vi "Day of the Week Predictor.vi"(6 "EXIT":bool, 7 "Guess the Day":bool, 8 "error in":errorcluster, 9 "YEAR\n(0-2399)A.D":i32, 10 "DATE":u16(ring) items=["1", "2", "3", "4", "5", "6", "7", "8", "9", "10", "11", "12", "13", "14", "15", "16", "17", "18", "19", "20", "21", "22", "23", "24", "25", "26", "27", "28", "29", "30", "31"], 11 "MONTH":T1(ring)) -> (0 "error out":errorcluster)   [LabVIEW 2020]
doc: "This VI will predict the Day of the Week from a given set of years (0-2399) A.D.\nUser can set the Month,Date,Year and then Click the \"GUESS THE DAY\" button to get the Day from given details."
uses:
  <vilib>/regexp/Match Regular Expression.xnode
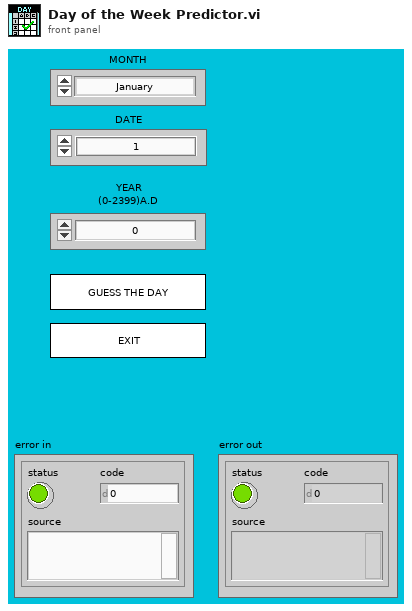
[diagram p1: front panel]
types:
  T1 = enum16{"January", "February", "March", "April", "May", "June", "July", "August", "September", "October", "November", "December"}
  T2 = enum32{"Invalid", "Standard", "Closed", "Hidden", "Minimized", "Maximized"}
  T3 = enum32{"invalid app kind", "Development System", "Run Time System", "Student Edition", "Embedded LabVIEW", "Evaluation", "Custom"}
  T4 = cluster{"Core":cluster{"Current VI Reference":refnum<vi>, "Close Panel on Exit?":bool}, "Your Boolean data":bool, "Your string data":string, "Year":i32, "Month":enum16{"January", "February", "March", "April", "May", "June", "July", "August", "September", "October", "November", "December"}, "Date":enum16{"1", "2", "3", "4", "5", "6", "7", "8", "9", "10", "11", "12", "13", "14", "15", "16", "17", "18", "19", "20", "21", "22", "23", "24", "25", "26", "27", "28", "29", "30", "31"}, "Last two Digits(Year)":i32, "Quotient(/4)":i32, "Month Code":i32, "Year Code":i32}
  T5 = enum16{"1", "2", "3", "4", "5", "6", "7", "8", "9", "10", "11", "12", "13", "14", "15", "16", "17", "18", "19", "20", "21", "22", "23", "24", "25", "26", "27", "28", "29", "30", "31"}
  T6 = cluster{"Current VI Reference":refnum<vi>, "Close Panel on Exit?":bool}
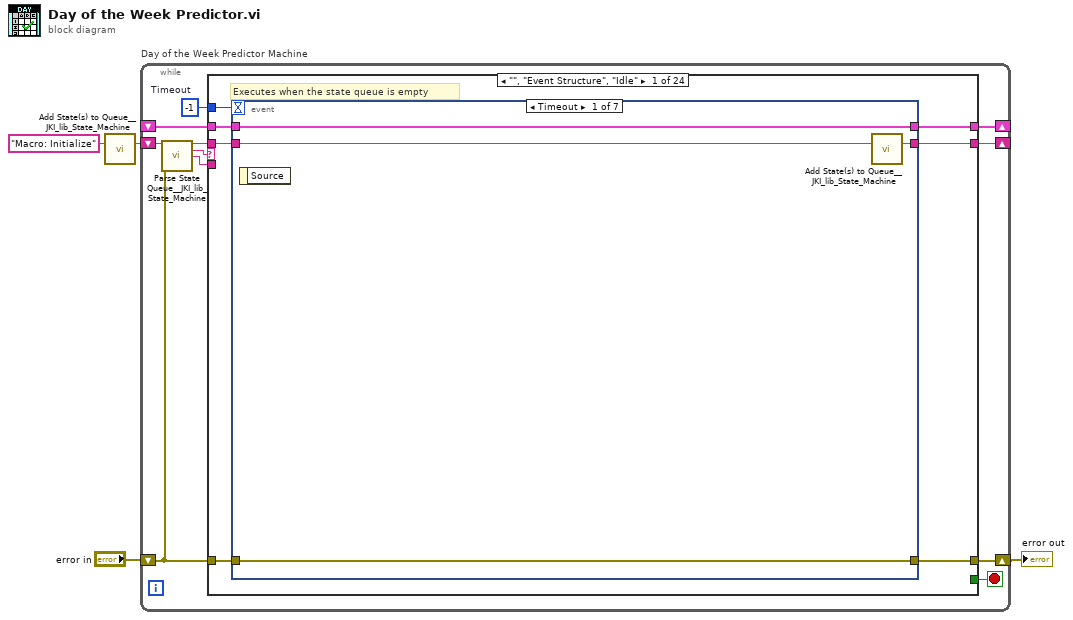
[diagram p0: block diagram]
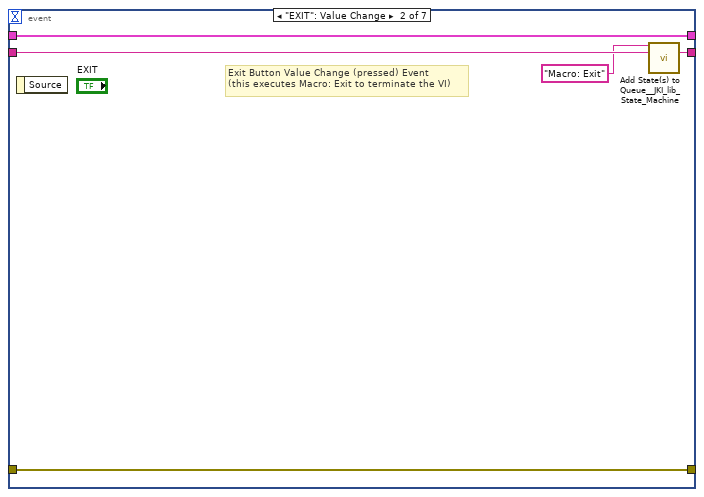
[diagram p2: hidden frame]
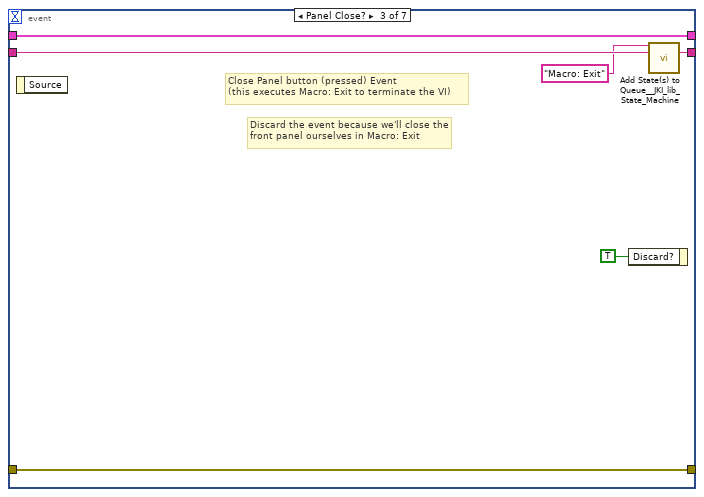
[diagram p3: hidden frame]
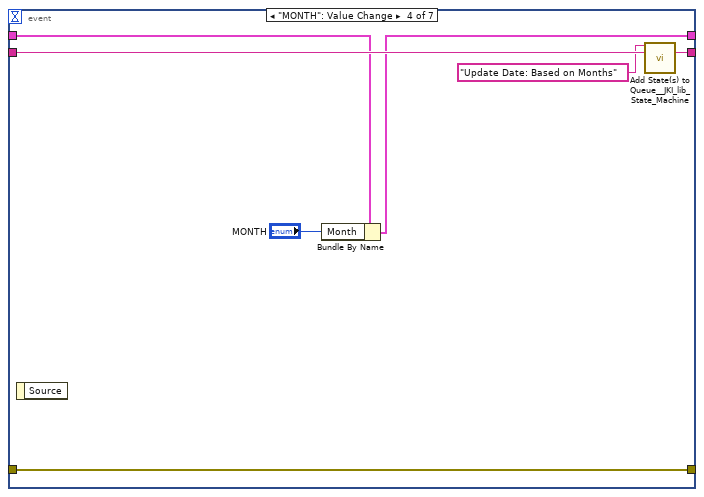
[diagram p4: hidden frame]
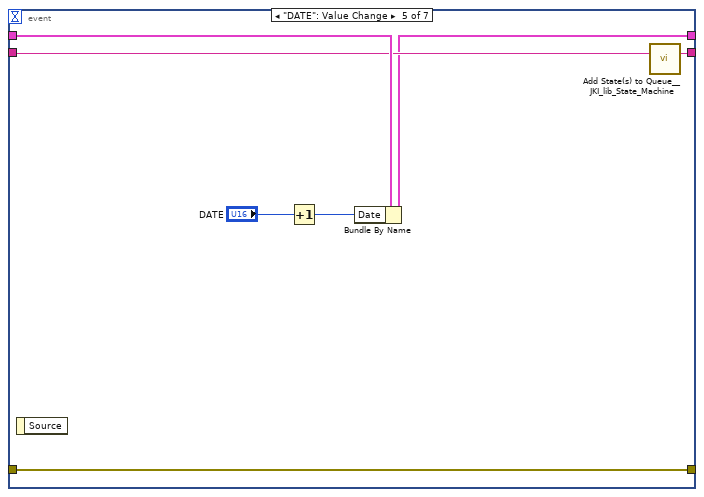
[diagram p5: hidden frame]
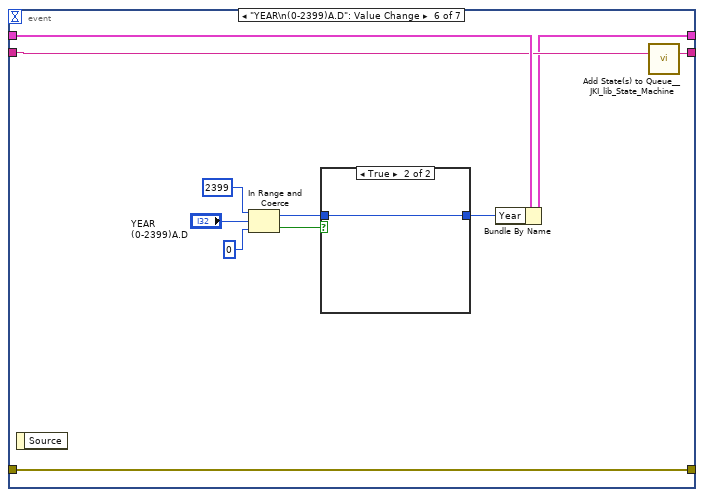
[diagram p6: hidden frame]
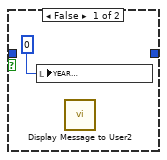
[diagram p7: hidden frame]
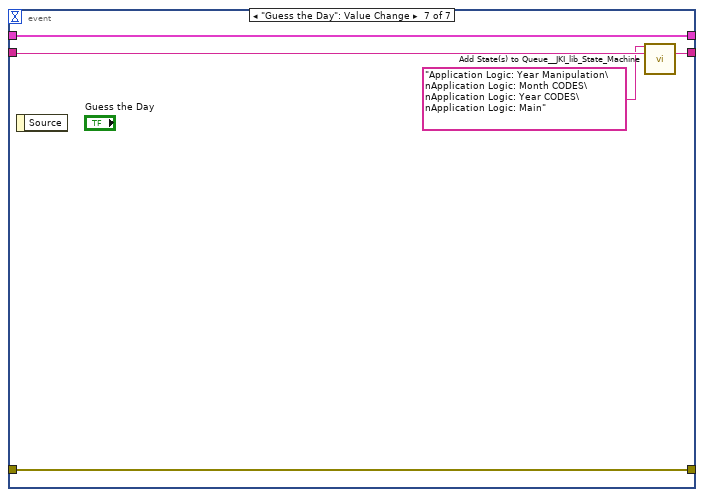
[diagram p8: hidden frame]
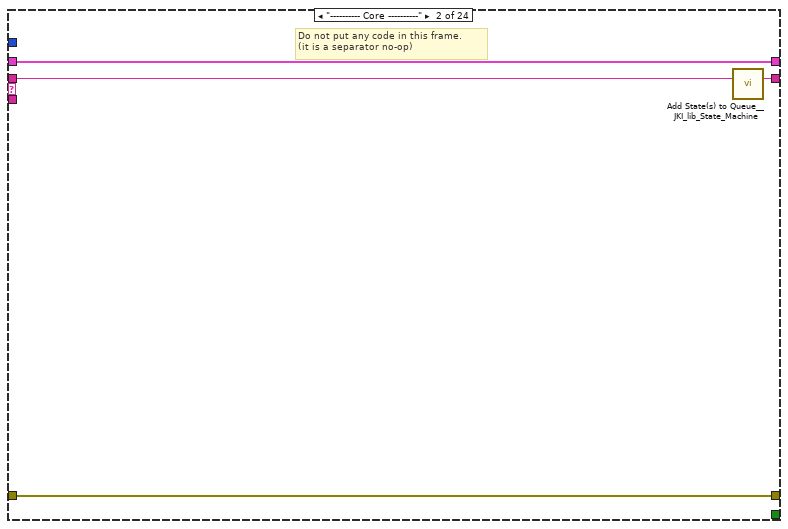
[diagram p9: hidden frame]
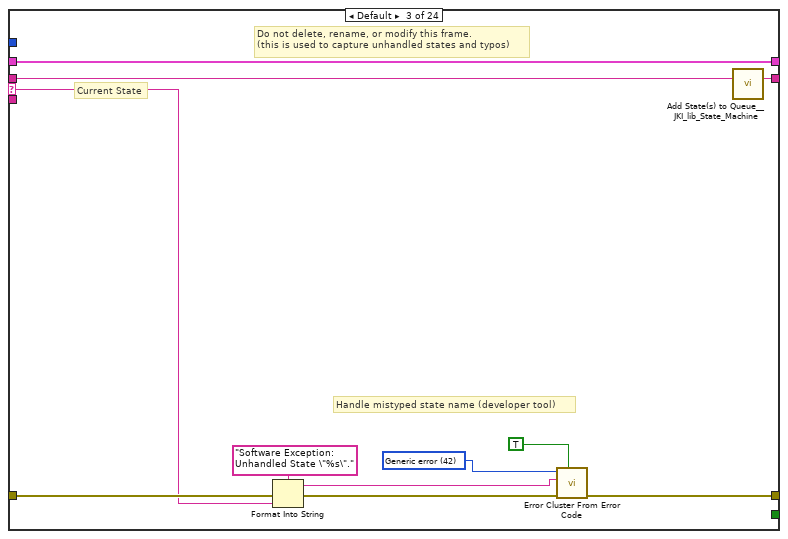
[diagram p10: hidden frame]
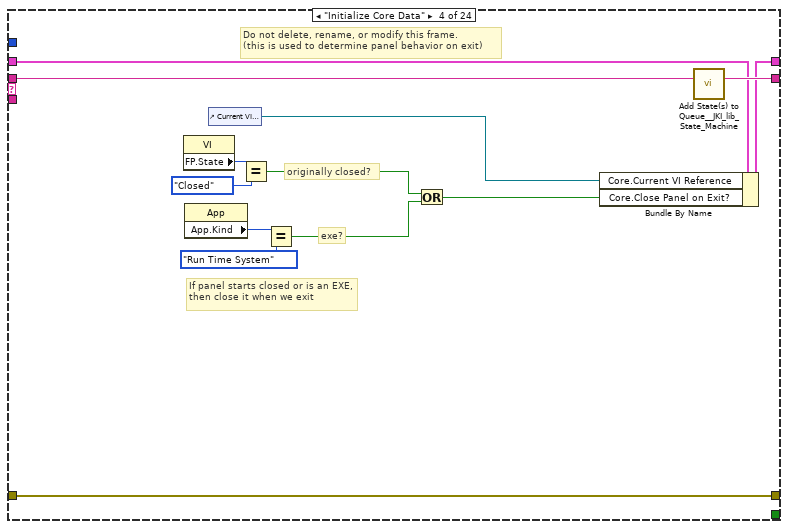
[diagram p11: hidden frame]
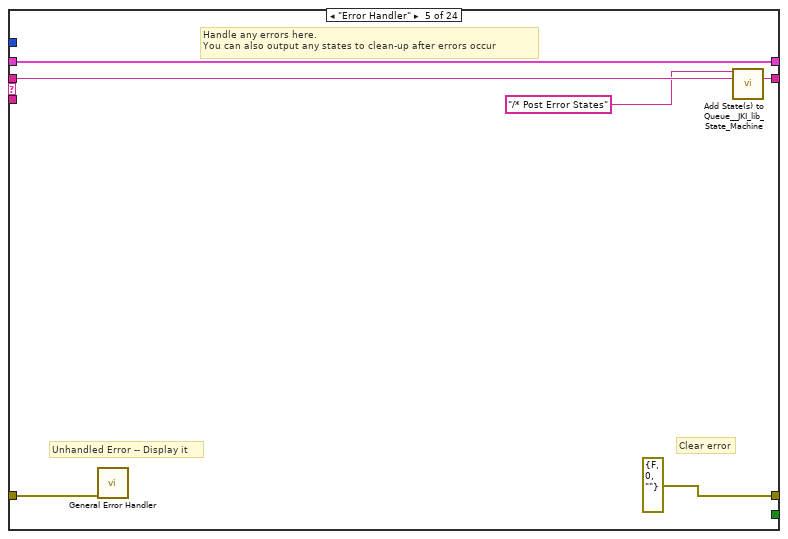
[diagram p12: hidden frame]
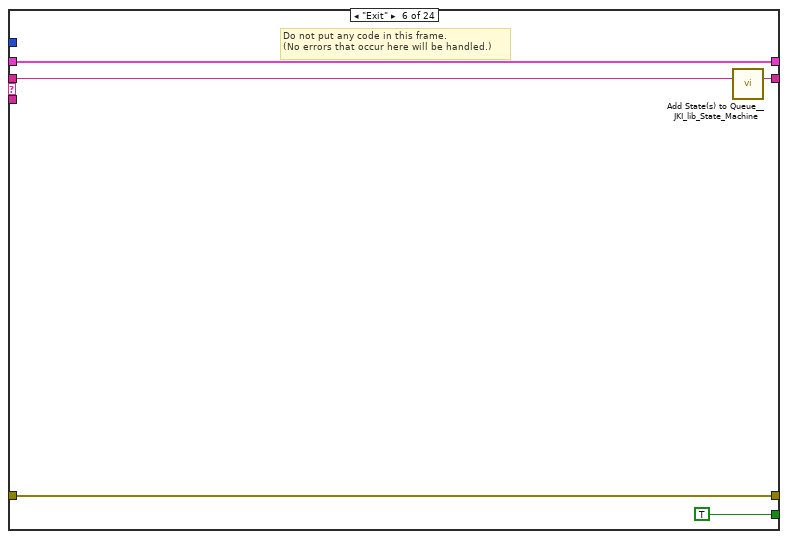
[diagram p13: hidden frame]
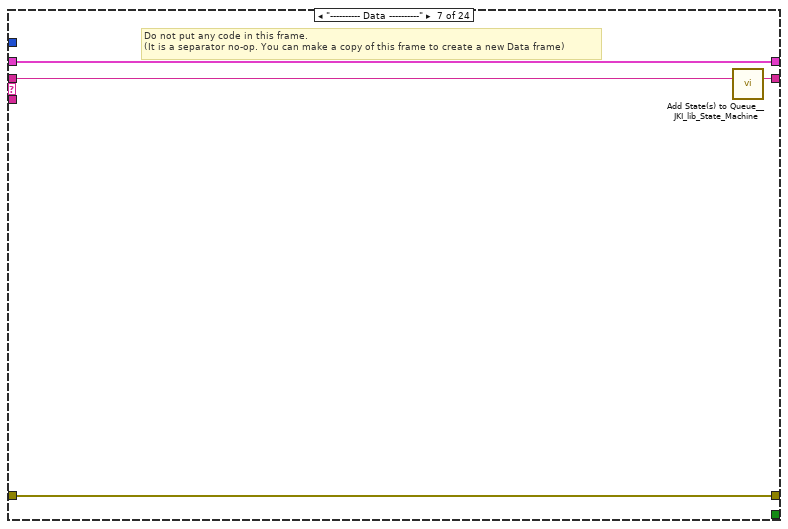
[diagram p14: hidden frame]
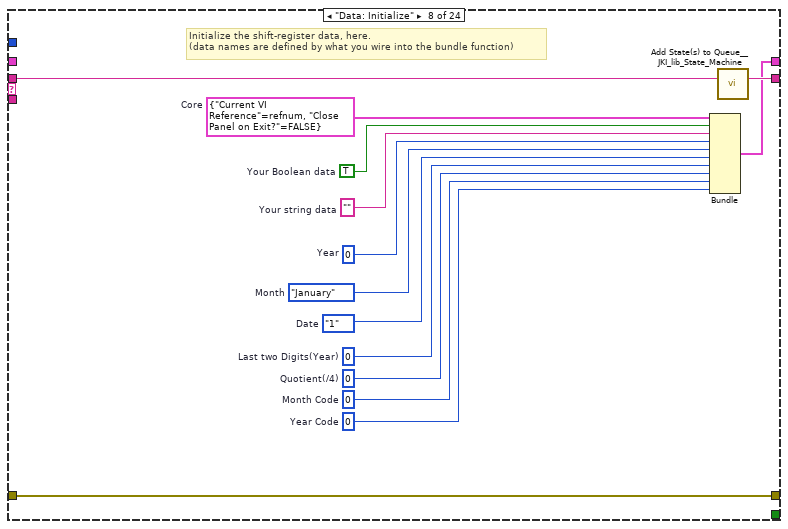
[diagram p15: hidden frame]
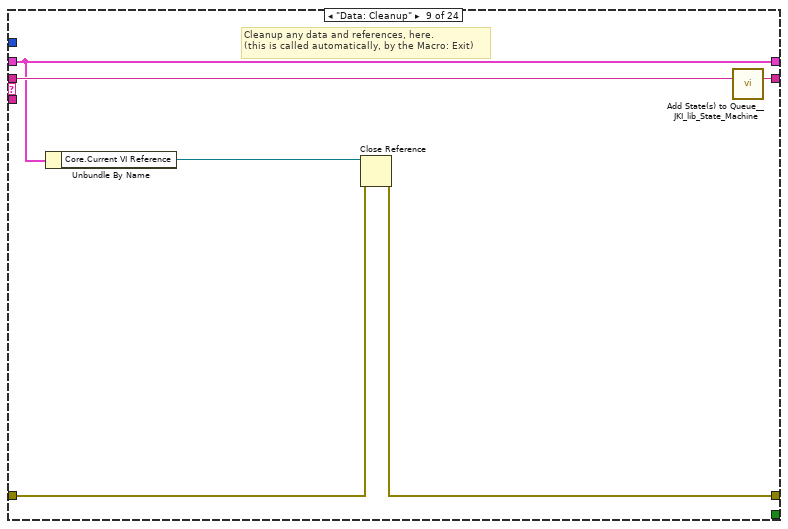
[diagram p16: hidden frame]
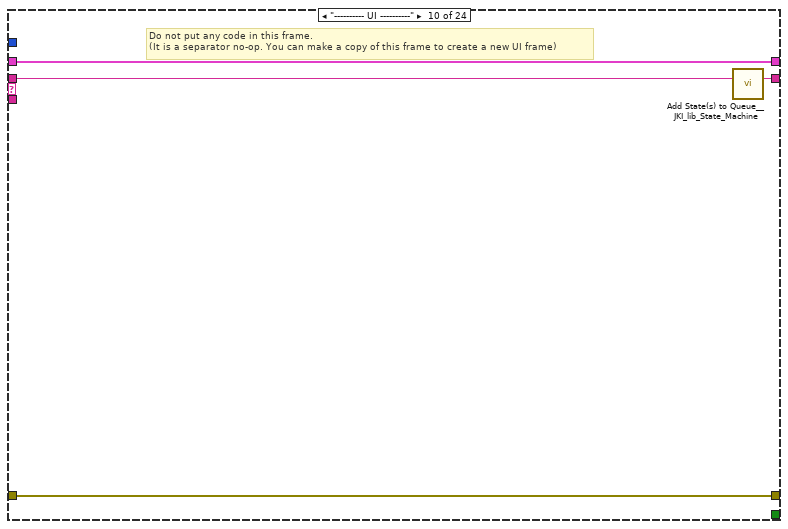
[diagram p17: hidden frame]
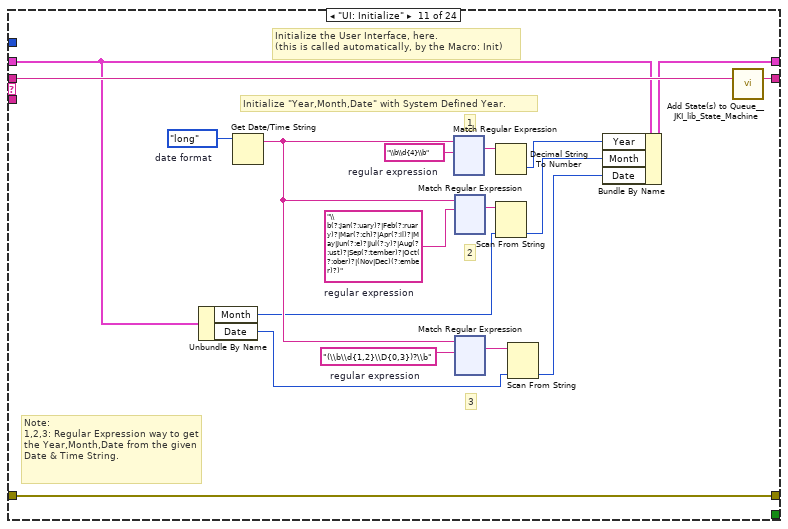
[diagram p18: hidden frame]
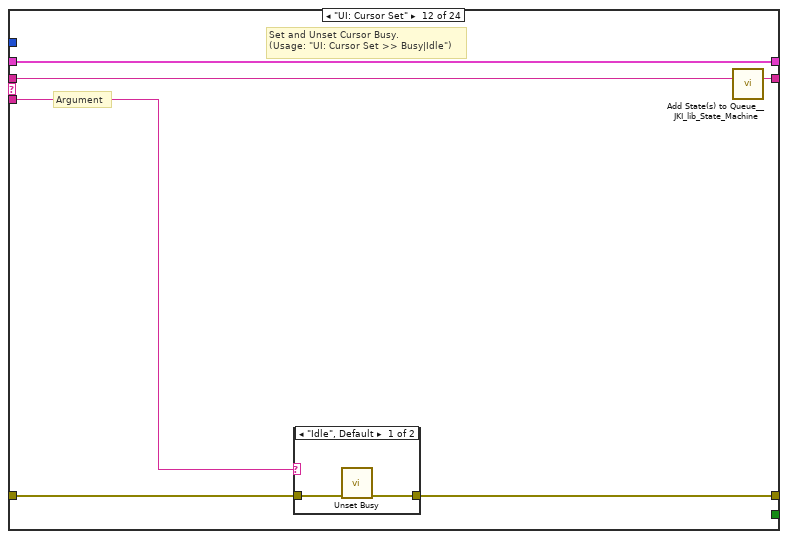
[diagram p19: hidden frame]
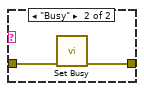
[diagram p20: hidden frame]
diagram:
  n1 = call <vilib>:"Add State(s) to Queue__JKI_lib_State_Machine.vi"("State(s) in (\"\")"="Macro: Initialize") -> ("States Out"=w4:string)  [unwired: 14 in]
  n2 = while "Day of the Week Predictor Machine" {
    shift-right: [w8] -> _
    shift-left: _ -> [w7]
    shift-right: [w11] -> w1
    shift-left: "error in" -> [w5]
    shift-right: [w10] -> _
    shift-left: w4 -> [w12]
    stop <- w9 stop-if-true
    w6 = -1  # Timeout
    n3 = call <vilib>:"Parse State Queue__JKI_lib_State_Machine.vi"("State Queue"=w12, "Error In (no error)"=w5) -> ("Remaining States"=w14:string, "Current State"=w15:string, "Arguments"=w13:string)  [unwired: 11 in]
    n4 = case shown="\"\", \"Event Structure\", \"Idle\"" w15 {
      selector: w15 -> [_ _ w74 _ _ _ _ _ _ _ _ _ _ _ _ _ _ _ _ _ _ _ _ _]
      tunnel: w14 -> [w22 w73 w78 w97 w103 w108 w112 w126 w132 w136 w154 w502 w513 w585 w589 w594 w604 w608 w616 w632 w645 w663 w670 w690]
      tunnel: w13 -> [_ _ _ _ _ _ _ _ _ _ _ w497 w507 _ _ _ _ _ _ _ _ _ _ _]
      tunnel: w7 -> [w20 w70 w76 w90 w100 w106 w109 _ w127 w133 w140 w500 w509 w582 w586 w591 w601 w605 w613 w629 w642 w660 w667 w687]
      tunnel: [w19 w71 w80 w94 errorcluster {"status"=FALSE, "code"=0, "source"=""} ("error out") w105 w110 w123 w128 w134 w152 w498 w510 w583 w587 w592 w602 w606 w614 w630 w643 w661 w668 w688] -> w11
      tunnel: w5 -> [w18 w71 w79 w94 w99 w105 w110 w123 w129 w134 w152 w499 w511 w583 w587 w592 w602 w606 w614 w630 w643 w661 w668 w688]
      tunnel: [w21 w72 w77 w96 w102 w107 w111 w125 w131 w135 w153 w501 w512 w584 w588 w593 w603 w607 w615 w631 w644 w662 w669 w689] -> w10
      tunnel: [_ _ _ _ _ TRUE _ _ _ _ _ _ _ _ _ _ _ _ _ _ _ _ _ _] -> w9
      tunnel: [w17 w70 w76 w95 w100 w106 w109 w124 w127 w133 w148 w500 w509 w582 w586 w591 w601 w605 w613 w629 w642 w656 w665 w685] -> w8
      tunnel: w6 -> [w16 _ _ _ _ _ _ _ _ _ _ _ _ _ _ _ _ _ _ _ _ _ _ _]
      frame "", "Event Structure", "Idle" {
        # "Executes when the state queue is empty"
        n5 = event shown="[0] Timeout" {
          selector: _ -> [_ _ _ _ _ _ _]
          dyn-events: _ -> [_ _ _ _ _ _ _]
          timeout: w16 -> [_ _ _ _ _ _ _]
          tunnel: w22 -> [w26 w31 w37 w43 w49 w59 w66]
          tunnel: [w25 w30 w36 w44 w50 w60 w67] -> w21
          tunnel: w20 -> [w23 w28 w34 w41 w51 w62 w68]
          tunnel: [w24 w29 w35 w38 w47 w61 w69] -> w19
          tunnel: w18 -> [w24 w29 w35 w38 w47 w61 w69]
          tunnel: [w23 w28 w34 w40 w48 w58 w68] -> w17
          event Timeout {
            n6 = event-data() -> ()  [unwired: 1 in, 1 out]
            n7 = call <vilib>:"Add State(s) to Queue__JKI_lib_State_Machine.vi"("State(s) in (\"\")"=w26) -> ("States Out"=w25:string)  [unwired: 14 in]
          }
          event "EXIT": Value Change {
            # "Exit Button Value Change (pressed) Event\n(this executes Macro: Exit to terminate the VI)"
            n8 = event-data() -> ()  [unwired: 1 in, 1 out]
            n9 = call <vilib>:"Add State(s) to Queue__JKI_lib_State_Machine.vi"("State(s) in Front (\"\")"="Macro: Exit", "State(s) in (\"\")"=w31) -> ("States Out"=w30:string)  [unwired: 13 in]
          }
          event Panel Close? {
            # "Discard the event because we'll close the front panel ourselves in Macro: Exit"
            # "Close Panel button (pressed) Event\n(this executes Macro: Exit to terminate the VI)"
            n10 = event-data() -> ()  [unwired: 1 in, 1 out]
            n11 = event-data("Discard?"=TRUE) -> ()  [unwired: 1 in, 1 out]
            n12 = call <vilib>:"Add State(s) to Queue__JKI_lib_State_Machine.vi"("State(s) in Front (\"\")"="Macro: Exit", "State(s) in (\"\")"=w37) -> ("States Out"=w36:string)  [unwired: 13 in]
          }
          event "MONTH": Value Change {
            n13 = event-data() -> ()  [unwired: 1 in, 1 out]
            n14 = Bundle By Name(cluster=w41, "Month"="MONTH") -> (w40:T4)
            n15 = call <vilib>:"Add State(s) to Queue__JKI_lib_State_Machine.vi"("State(s) in Front (\"\")"="Update Date: Based on Months", "State(s) in (\"\")"=w43) -> ("States Out"=w44:string)  [unwired: 13 in]
          }
          event "DATE": Value Change {
            n16 = event-data() -> ()  [unwired: 1 in, 1 out]
            n17 = Increment(x="DATE") -> (x+1=w45:u16)
            n18 = Bundle By Name(cluster=w51, "Date"=w45) -> (w48:T4)
            n19 = call <vilib>:"Add State(s) to Queue__JKI_lib_State_Machine.vi"("State(s) in (\"\")"=w49) -> ("States Out"=w50:string)  [unwired: 14 in]
          }
          event "YEAR\n(0-2399)A.D": Value Change {
            n20 = event-data() -> ()  [unwired: 1 in, 1 out]
            n21 = In Range and Coerce(upper limit=2399, x="YEAR\n(0-2399)A.D", lower limit=0) -> (coerced(x)=w53:i32, In Range?=w54:bool)
            n22 = case shown="True" w54 {
              tunnel: [_ w64] -> w52
              tunnel: w53 -> [_ w64]
              frame False {
                n23 = local write "YEAR\n(0-2399)A.D"(0 ("YEAR\n(0-2399)A.D")) -> ()
                n24 = call "Display Message to User2"() -> ()  [unwired: 10 in, 2 out]
              }
              frame True {
              }
            }
            n25 = Bundle By Name(cluster=w62, "Year"=w52) -> (w58:T4)
            n26 = call <vilib>:"Add State(s) to Queue__JKI_lib_State_Machine.vi"("State(s) in (\"\")"=w59) -> ("States Out"=w60:string)  [unwired: 14 in]
          }
          event "Guess the Day": Value Change {
            n27 = event-data() -> ()  [unwired: 1 in, 1 out]
            n28 = call <vilib>:"Add State(s) to Queue__JKI_lib_State_Machine.vi"("State(s) in Front (\"\")"="Application Logic: Year Manipulation\nApplication Logic: Month CODES\nApplication Logic: Year CODES\nApplication Logic: Main" ("State(s) in (\"\")"), "State(s) in (\"\")"=w66) -> ("States Out"=w67:string)  [unwired: 13 in]
          }
        }
      }
      frame "---------- Core ----------" {
        # "Do not put any code in this frame.\n(it is a separator no-op)"
        n29 = call <vilib>:"Add State(s) to Queue__JKI_lib_State_Machine.vi"("State(s) in (\"\")"=w73) -> ("States Out"=w72:string)  [unwired: 14 in]
      }
      frame Default {
        w83 = 42 items=["No error", "Argument error", "Memory is full", "Out of zone", "End of file", "File already open", "Generic file I/O error", "File not found", "File permission error", "Disk is full", "Duplicate path", "Too many files open", "System feature not enabled", "Resource file not found", "Cannot add resource", "Resource not found", "Image not found", "Image memory error", "Pen does not exist", "Config type invalid", "Config token not found", "Config parse error", "Config memory error", "Bad external code format", "Bad external code offset", "External code not present", "Null window", "Destroy window error", "Null menu", "Print aborted", "Bad print record", "Print driver error", "Windows error during printing", "Memory error during printing", "Print dialog error", "Generic print error", "Invalid device refnum", "Device not found", "Device parameter error", "Device unit error", "Cannot open device", "Device call aborted", "Generic error", "Cancelled by user", "Object ID too low", "Object ID too high", "Object not in heap", "Unknown heap", "Unknown object (invalid DefProc)", "Unknown object (DefProc not in table)", "Message out of range", "Invalid (null) method", "Unknown message", "Manager call not supported", "Bad address", "Network operation in progress", "Network operation timed out", "Connection is busy", "Network attribute not supported", "Network error", "Address in use", "System out of memory", "Connection aborted", "Connection refused", "Not connected", "Already connected", "Connection closed", "Initialization error (interapplication manager)", "Bad occurrence", "Wait on unbound occurrence handler", "Occurrence queue overflow", "Datalog type conflict", "Unused", "Unrecognized type (interapplication manager)", "Memory corrupt", "Failed to make temporary DLL", "Old CIN version", "Drag socket not found", "Failed to load drop-object", "Failed to register OLE object", "Failed to release OLE object", "Format specifier type mismatch", "Unknown format specifier", "Too few format specifiers", "Too many format specifiers", "Scan failed", "Newer CIN version", "Error converting to variant", "Runtime menu error", "Password tampered", "Variant attribute not found", "Incompatible variant data type", "Event data is not available", "Event Store is not present", "Occurrence is not found", "Event Queue is not created", "Event info is not available", "Refnum passed is NULL", "Error retrieving Class GUID", "Error retrieving CoClass GUID", "Error retrieving TypeLib GUID.", "Bad built application magic bytes.", "Specific driver is different from the specific driver associated with the Logical Name.", "There is no session opened to the class driver.", "Max Error", "MAX - Error with config objects", "MAX - Error loading configuration", "MAX - Group not supported"]
        # "Current State"
        # "Do not delete, rename, or modify this frame.\n(this is used to capture unhandled states and typos)"
        # "Handle mistyped state name (developer tool)"
        n30 = Format Into String(format string="Software Exception: Unhandled State \"%s\"." ("message"), error in=w79, w74) -> (resulting string=w82:string, error out=w81:errorcluster)  [unwired: 1 in]
        n31 = call <vilib>:"Error Cluster From Error Code.vi"("show call chain? (False)"=TRUE, "error in (no error)"=w81, "error message (\"\")"=w82, "error code (0)"=w83) -> ("error out"=w80:errorcluster)  [unwired: 5 in]
        n32 = call <vilib>:"Add State(s) to Queue__JKI_lib_State_Machine.vi"("State(s) in (\"\")"=w78) -> ("States Out"=w77:string)  [unwired: 14 in]
      }
      frame "Initialize Core Data" {
        # "Do not delete, rename, or modify this frame.\n(this is used to determine panel behavior on exit)"
        # "originally closed?"
        # "exe?"
        # "If panel starts closed or is an EXE, then close it when we exit"
        n33 = property class="VI"() -> ("FP.State"=w87:T2)  [unwired: 2 in, 2 out]
        n34 = property class="App"() -> ("App.Kind"=w93:T3)  [unwired: 2 in, 2 out]
        n35 = control-ref of="Current VI Reference"() -> (w88:refnum<vi>)
        n36 = Equal?(x=w87, y=T2."Closed" ("Front Panel Window:State")) -> (x = y?=w85:bool)
        n37 = Equal?(x=w93, y=T3."Run Time System" ("Application:Kind")) -> (x = y?=w91:bool)
        n38 = Or(x=w85, y=w91) -> (x .or. y?=w89:bool)
        n39 = Bundle By Name(cluster=w90, "Core.Current VI Reference"=w88, "Core.Close Panel on Exit?"=w89) -> (w95:T4)
        n40 = call <vilib>:"Add State(s) to Queue__JKI_lib_State_Machine.vi"("State(s) in (\"\")"=w97) -> ("States Out"=w96:string)  [unwired: 14 in]
      }
      frame "Error Handler" {
        # "Unhandled Error -- Display it"
        # "Handle any errors here.\nYou can also output any states to clean-up after errors occur"
        # "Clear error"
        n41 = call <vilib>:"General Error Handler.vi"("error in (no error)"=w99) -> ()  [unwired: 10 in, 5 out]
        n42 = call <vilib>:"Add State(s) to Queue__JKI_lib_State_Machine.vi"("State(s) in Front (\"\")"="/* Post Error States", "State(s) in (\"\")"=w103) -> ("States Out"=w102:string)  [unwired: 13 in]
      }
      frame "Exit" {
        # "Do not put any code in this frame.\n(No errors that occur here will be handled.)"
        n43 = call <vilib>:"Add State(s) to Queue__JKI_lib_State_Machine.vi"("State(s) in (\"\")"=w108) -> ("States Out"=w107:string)  [unwired: 14 in]
      }
      frame "---------- Data ----------" {
        # "Do not put any code in this frame.\n(It is a separator no-op. You can make a copy of this frame to create a new Data frame)"
        n44 = call <vilib>:"Add State(s) to Queue__JKI_lib_State_Machine.vi"("State(s) in (\"\")"=w112) -> ("States Out"=w111:string)  [unwired: 14 in]
      }
      frame "Data: Initialize" {
        w113 = 0  # Year Code
        w114 = 0  # Month Code
        w115 = 0  # Quotient(/4)
        w116 = 0  # Last two Digits(Year)
        w117 = T5."1"  # Date
        w118 = T1."January"  # Month
        w119 = 0  # Year
        w120 = T6 {"Current VI Reference"=refnum, "Close Panel on Exit?"=FALSE}  # Core
        w122 = TRUE  # Your Boolean data
        w121 = ""  # Your string data
        # "Initialize the shift-register data, here.\n(data names are defined by what you wire into the bundle function)"
        n45 = Bundle("Core"=w120, "Your Boolean data"=w122, "Your string data"=w121, "Year"=w119, "Month"=w118, "Date"=w117, "Last two Digits(Year)"=w116, "Quotient(/4)"=w115, "Month Code"=w114, "Year Code"=w113) -> (w124:T4)  [unwired: 1 in]
        n46 = call <vilib>:"Add State(s) to Queue__JKI_lib_State_Machine.vi"("State(s) in (\"\")"=w126) -> ("States Out"=w125:string)  [unwired: 14 in]
      }
      frame "Data: Cleanup" {
        # "Cleanup any data and references, here.\n(this is called automatically, by the Macro: Exit)"
        n47 = Unbundle By Name(w127) -> ("Core.Current VI Reference"=w130:refnum<vi>)
        n48 = Close Reference(reference=w130, error in (no error)=w129) -> (error out=w128:errorcluster)
        n49 = call <vilib>:"Add State(s) to Queue__JKI_lib_State_Machine.vi"("State(s) in (\"\")"=w132) -> ("States Out"=w131:string)  [unwired: 14 in]
      }
      frame "---------- UI ----------" {
        # "Do not put any code in this frame.\n(It is a separator no-op. You can make a copy of this frame to create a new UI frame)"
        n50 = call <vilib>:"Add State(s) to Queue__JKI_lib_State_Machine.vi"("State(s) in (\"\")"=w136) -> ("States Out"=w135:string)  [unwired: 14 in]
      }
      frame "UI: Initialize" {
        w143 = "(\\b\\d{1,2}\\D{0,3})?\\b"  # regular expression
        w145 = "\\b(?:Jan(?:uary)?|Feb(?:ruary)?|Mar(?:ch)?|Apr(?:il)?|May|Jun(?:e)?|Jul(?:y)?|Aug(?:ust)?|Sep(?:tember)?|Oct(?:ober)?|(Nov|Dec)(?:ember)?)"  # regular expression
        w149 = "\\b\\d{4}\\b"  # regular expression
        w151 = enum16{"short", "long", "abbreviated"}."long"  # date format
        # "Note:\n1,2,3: Regular Expression way to get the Year,Month,Date from the given Date & Time String."
        # "3"
        # "2"
        # "1"
        # "Initialize \"Year,Month,Date\" with System Defined Year."
        # "Initialize the User Interface, here.\n(this is called automatically, by the Macro: Init)"
        n51 = Unbundle By Name(w140) -> ("Month"=w139:T1, "Date"=w138:T5)
        n52 = Get Date/Time String(date format (0)=w151) -> (date string=w144:string)  [unwired: 2 in, 1 out]
        n53 = xnode ("Match Regular Expression")("input string"=w144, "regular expression"=w149) -> ("whole match"=w150:string)  [unwired: 4 in, 4 out]
        n54 = xnode ("Match Regular Expression")("input string"=w144, "regular expression"=w145) -> ("whole match"=w146:string)  [unwired: 4 in, 4 out]
        n55 = xnode ("Match Regular Expression")("input string"=w144, "regular expression"=w143) -> ("whole match"=w141:string)  [unwired: 4 in, 4 out]
        n56 = Decimal String To Number(string=w150) -> (number=w147:i32)  [unwired: 2 in, 1 out]
        n57 = Scan From String(input string=w146, default 1=w139) -> (output 1=w142:T1)  [unwired: 3 in, 3 out]
        n58 = Scan From String(input string=w141, default 1=w138) -> (output 1=w137:T5)  [unwired: 3 in, 3 out]
        n59 = Bundle By Name(cluster=w140, "Year"=w147, "Month"=w142, "Date"=w137) -> (w148:T4)
        n60 = call <vilib>:"Add State(s) to Queue__JKI_lib_State_Machine.vi"("State(s) in (\"\")"=w154) -> ("States Out"=w153:string)  [unwired: 14 in]
      }
      frame "UI: Cursor Set" {
        # "Argument"
        # "Set and Unset Cursor Busy.\n(Usage: \"UI: Cursor Set >> Busy|Idle\")"
        n61 = case shown="\"Idle\", Default" w497 {
          tunnel: w499 -> [w504 w506]
          tunnel: [w503 w505] -> w498
          frame "Idle", Default {
            n62 = call <vilib>:"Unset Busy.vi"("error in (no error)"=w504) -> ("error out"=w503:errorcluster)  [unwired: 10 in]
          }
          frame "Busy" {
            n63 = call <vilib>:"Set Busy.vi"("error in (no error)"=w506) -> ("error out"=w505:errorcluster)  [unwired: 9 in, 1 out]
          }
        }
        n64 = call <vilib>:"Add State(s) to Queue__JKI_lib_State_Machine.vi"("State(s) in (\"\")"=w502) -> ("States Out"=w501:string)  [unwired: 14 in]
      }
      frame "UI: Front Panel State" {
        # "Argument"
        # "Set Front Panel Open or Closed\n(Usage: \"UI: Front Panel State >> Open|Close\")"
        n65 = Unbundle By Name(w509) -> ("Core.Current VI Reference"=w508:refnum<vi>)
        n66 = case shown="\"Open\", \"Standard\", Default" w507 {
          tunnel: w511 -> [w519 w534 w545 w558 w571]
          tunnel: [w521 w535 w547 w560 w573] -> w510
          tunnel: w508 -> [w520 w532 w546 w559 w572]
          frame "Open", "Standard", Default {
            w514 = T2."Standard" ("State")
            n67 = property class="VI"(reference=w520, error in=w519) -> (reference out=w517:refnum<vi>, error out=w518:errorcluster, "FP.State"=w516:T2)
            n68 = Not Equal?(x=w516, y=w514) -> (x != y?=w515:bool)
            n69 = case shown="False" w515 {
              tunnel: [w525 w527] -> w521
              tunnel: w518 -> [w524 w527]
              tunnel: w517 -> [w523 _]
              tunnel: w514 -> [w522 _]
              frame True {
                n70 = invoke class="VI" method="FP.Open"(reference=w523, error in=w524, "Activate"=TRUE, "State"=w522) -> (error out=w525:errorcluster)  [unwired: 1 in, 4 out]
              }
              frame False {
              }
            }
          }
          frame "Close", "Closed" {
            n71 = property class="VI"(reference=w532, error in=w534) -> (reference out=w531:refnum<vi>, error out=w533:errorcluster, "FP.State"=w529:T2)
            n72 = Not Equal?(x=w529, y=T2."Closed" ("Front Panel Window:State")) -> (x != y?=w528:bool)
            n73 = case shown="True" w528 {
              tunnel: [w536 w539] -> w535
              tunnel: w533 -> [w536 w538]
              tunnel: w531 -> [_ w537]
              frame False {
              }
              frame True {
                n74 = invoke class="VI" method="FP.Close"(reference=w537, error in=w538) -> (error out=w539:errorcluster)  [unwired: 1 in, 2 out]
              }
            }
          }
          frame "Hidden", "Hide" {
            w540 = T2."Hidden" ("State")
            n75 = property class="VI"(reference=w546, error in=w545) -> (reference out=w543:refnum<vi>, error out=w544:errorcluster, "FP.State"=w542:T2)
            n76 = Not Equal?(x=w542, y=w540) -> (x != y?=w541:bool)
            n77 = case shown="True" w541 {
              tunnel: [w551 w552] -> w547
              tunnel: w544 -> [w550 w552]
              tunnel: w543 -> [w549 _]
              tunnel: w540 -> [w548 _]
              frame True {
                n78 = invoke class="VI" method="FP.Open"(reference=w549, error in=w550, "State"=w548) -> (error out=w551:errorcluster)  [unwired: 2 in, 4 out]
              }
              frame False {
              }
            }
          }
          frame "Minimize", "Minimized" {
            w553 = T2."Minimized" ("State")
            n79 = property class="VI"(reference=w559, error in=w558) -> (reference out=w556:refnum<vi>, error out=w557:errorcluster, "FP.State"=w555:T2)
            n80 = Not Equal?(x=w555, y=w553) -> (x != y?=w554:bool)
            n81 = case shown="True" w554 {
              tunnel: [w564 w565] -> w560
              tunnel: w557 -> [w563 w565]
              tunnel: w556 -> [w562 _]
              tunnel: w553 -> [w561 _]
              frame True {
                n82 = invoke class="VI" method="FP.Open"(reference=w562, error in=w563, "State"=w561) -> (error out=w564:errorcluster)  [unwired: 2 in, 4 out]
              }
              frame False {
              }
            }
          }
          frame "Maximize", "Maximized" {
            w566 = T2."Maximized" ("State")
            n83 = property class="VI"(reference=w572, error in=w571) -> (reference out=w569:refnum<vi>, error out=w570:errorcluster, "FP.State"=w568:T2)
            n84 = Not Equal?(x=w568, y=w566) -> (x != y?=w567:bool)
            n85 = case shown="True" w567 {
              tunnel: [w577 w578] -> w573
              tunnel: w570 -> [w576 w578]
              tunnel: w569 -> [w575 _]
              tunnel: w566 -> [w574 _]
              frame True {
                n86 = invoke class="VI" method="FP.Open"(reference=w575, error in=w576, "State"=w574) -> (error out=w577:errorcluster)  [unwired: 2 in, 4 out]
              }
              frame False {
              }
            }
          }
        }
        n87 = call <vilib>:"Add State(s) to Queue__JKI_lib_State_Machine.vi"("State(s) in (\"\")"=w513) -> ("States Out"=w512:string)  [unwired: 14 in]
      }
      frame "UI: Update" {
        # "Updates the User Interface!\n(Front Panel Objects are updated here in this State)"
        n88 = Unbundle By Name(w582) -> ("Month"=w581:T1, "Date"=w579:T5, "Year"=w580:i32)
        n89 = local write "YEAR\n(0-2399)A.D"(w580) -> ()
        n90 = local write "MONTH"(w581) -> ()
        n91 = local write "DATE"(w579) -> ()
        n92 = call <vilib>:"Add State(s) to Queue__JKI_lib_State_Machine.vi"("State(s) in (\"\")"=w585) -> ("States Out"=w584:string)  [unwired: 14 in]
      }
      frame "---------- Macro ----------" {
        # "Do not put any code in this frame.\n(It is a separator no-op. You can make a copy of this frame to create a new Macro frame)"
        n93 = call <vilib>:"Add State(s) to Queue__JKI_lib_State_Machine.vi"("State(s) in (\"\")"=w589) -> ("States Out"=w588:string)  [unwired: 14 in]
      }
      frame "Macro: Initialize" {
        w590 = "Data: Initialize\nInitialize Core Data\nUI: Initialize\nUI: Update\nUI: Front Panel State >> Open"  # Data: Initialize Initialize Core Data UI: Initialize UI: Update UI: Front Panel State >> Open
        # "Initialization Macro\n(This is called once, when the VI starts)"
        n94 = call <vilib>:"Add State(s) to Queue__JKI_lib_State_Machine.vi"("State(s) in Front (\"\")"=w590, "State(s) in (\"\")"=w594) -> ("States Out"=w593:string)  [unwired: 13 in]
      }
      frame "Macro: Exit" {
        # "Exit Macro\n(This is called once, when the VI exits)"
        n95 = Unbundle By Name(w601) -> ("Core.Close Panel on Exit?"=w600:bool)
        n96 = Select(t="UI: Front Panel State >> Close", s=w600, f="") -> (s? t:f=w597:string)
        n97 = call <vilib>:"Add State(s) to Queue__JKI_lib_State_Machine.vi"("State(s) in (\"\")"=w597, "State(s) at Back (\"\")"="Data: Cleanup\nExit") -> ("States Out"=w595:string)  [unwired: 13 in]
        n98 = call <vilib>:"Add State(s) to Queue__JKI_lib_State_Machine.vi"("State(s) in Front (\"\")"=w595, "State(s) in (\"\")"=w604) -> ("States Out"=w603:string)  [unwired: 13 in]
      }
      frame "---------- Update Date ----------" {
        # "Template Separator\n(Do Not Insert any CODE HERE!)"
        n99 = call <vilib>:"Add State(s) to Queue__JKI_lib_State_Machine.vi"("State(s) in (\"\")"=w608) -> ("States Out"=w607:string)  [unwired: 14 in]
      }
      frame "Update Date: Based on Months" {
        # "Updates Date Enum!\n(Here the Date Number List is updated based upon the Month Selected by the USER)"
        n100 = Unbundle By Name(w613) -> ("Month"=w612:T1, "Year"=w611:i32)
        n101 = case shown="\"February\"" w612 {
          tunnel: w611 -> [_ _ w628]
          tunnel: [30 ("y") 31 ("y") w623] -> w610
          frame "April", "June", "September", "November" {
            # "Months with \"30\" number of Days."
          }
          frame "January", "March", "May", "July", "August", "October", "December" {
            # "Months with \"31\" number of Days."
          }
          frame "February" {
            # "Leap Year Check!"
            n102 = Quotient & Remainder(x=w628, y=4) -> (x-y*floor(x/y)=w622:i32)  [unwired: 1 out]
            n103 = Equal To 0?(x=w622) -> (x = 0?=w626:bool)
            n104 = Select(t=29 ("y"), s=w626, f=28 ("y")) -> (s? t:f=w623:i32)
          }
        }
        n105 = for {
          N: w610 -> [_]
          tunnel: [w617] -> w609 mode=indexing
          i -> [w619]
          # "To Update Date List!"
          n106 = Increment(x=w619) -> (x+1=w618:i32)
          n107 = Number To Decimal String "Number To \nDecimal String"(number=w618) -> (decimal integer string=w617:string)  [unwired: 1 in]
        }
        n108 = property on="DATE" class="Ring (strict)"("Strings []"=w609) -> ()  [unwired: 2 in, 2 out]
        n109 = call <vilib>:"Add State(s) to Queue__JKI_lib_State_Machine.vi"("State(s) in (\"\")"=w616) -> ("States Out"=w615:string)  [unwired: 14 in]
      }
      frame "---------- Application Logic ----------" {
        # "Template Separator\n(Do Not insert any CODE HERE!)"
        n110 = call <vilib>:"Add State(s) to Queue__JKI_lib_State_Machine.vi"("State(s) in (\"\")"=w632) -> ("States Out"=w631:string)  [unwired: 14 in]
      }
      frame "Application Logic: Main" {
        # "Day of the Week is predicted here!!\n(Logic to predict the DAY from the given Month,Year,Date is carried out here)"
        n111 = Unbundle By Name(w642) -> ("Last two Digits(Year)"=w641:i32, "Quotient(/4)"=w640:i32, "Date"=w639:T5, "Month Code"=w638:i32, "Year Code"=w637:i32)
        n112 = Compound Arithmetic op=ADD(w641, w640, w639, w638, w637) -> (w636:i32)
        n113 = Quotient & Remainder(x=w636, y=7) -> (x-y*floor(x/y)=w634:i32)  [unwired: 1 out]
        n114 = case "Which DAY?" shown="0" w634 {
          tunnel: ["Try Again!" "It's SUNDAY!" "It's MONDAY!" "It's TUESDAY!" "It's WEDNESDAY!" "It's THURSDAY!" "It's FRIDAY!" "It's SATURDAY!"] -> w633
          frame Default {
          }
          frame 0 {
          }
          frame 1 {
          }
          frame 2 {
          }
          frame 3 {
          }
          frame 4 {
          }
          frame 5 {
          }
          frame 6 {
          }
        }
        n115 = call "Display Message to User"("Message"=w633) -> ()  [unwired: 9 in, 2 out]
        n116 = call <vilib>:"Add State(s) to Queue__JKI_lib_State_Machine.vi"("State(s) in (\"\")"=w645) -> ("States Out"=w644:string)  [unwired: 14 in]
      }
      frame "Application Logic: Year Manipulation" {
        # "YEAR Data Manipulation!\n(Last two digits of the given year is taken out and it is divided by 4 where it's quotient is saved in the Data Cluster)"
        n117 = Unbundle By Name(w660) -> ("Year"=w659:i32)
        n118 = Quotient & Remainder(x=w659, y=100) -> (x-y*floor(x/y)=w654:i32)  [unwired: 1 out]
        n119 = Quotient & Remainder(x=w654, y=4) -> (floor(x/y)=w655:i32)  [unwired: 1 out]
        n120 = Bundle By Name(cluster=w660, "Last two Digits(Year)"=w654, "Quotient(/4)"=w655) -> (w656:T4)
        n121 = call <vilib>:"Add State(s) to Queue__JKI_lib_State_Machine.vi"("State(s) in (\"\")"=w663) -> ("States Out"=w662:string)  [unwired: 14 in]
      }
      frame "Application Logic: Month CODES" {
        # "Developer Defined Code!\n(Respective Codes are given to Each MONTH by the Developer of this Application.Please Do not modify this without the Developer Knowledge)"
        n122 = Unbundle By Name(w667) -> ("Month"=w666:T1)
        n123 = case "Month CODE?" shown="\"January\"" w666 {
          tunnel: [0 0 3 3 6 1 4 6 2 5 0 3 5] -> w664
          frame Default {
          }
          frame "January" {
          }
          frame "February" {
          }
          frame "March" {
          }
          frame "April" {
          }
          frame "May" {
          }
          frame "June" {
          }
          frame "July" {
          }
          frame "August" {
          }
          frame "September" {
          }
          frame "October" {
          }
          frame "November" {
          }
          frame "December" {
          }
        }
        n124 = Bundle By Name(cluster=w667, "Month Code"=w664) -> (w665:T4)
        n125 = call <vilib>:"Add State(s) to Queue__JKI_lib_State_Machine.vi"("State(s) in (\"\")"=w670) -> ("States Out"=w669:string)  [unwired: 14 in]
      }
      frame "Application Logic: Year CODES" {
        # "Developer Defined Code!\n(Respective Codes are given to a CENTURY by the Developer of this Application.Please Do not modify this without the Developer Knowledge)"
        n126 = Unbundle By Name(w687) -> ("Year"=w686:i32)
        n127 = case "Year CODE?" shown="2000..2099" w686 {
          tunnel: [0 6 4 2 0 6 4 2 0 6 4 2 0 6 4 2 0 6 4 2 0 6 4 2 0] -> w684
          frame Default {
          }
          frame 0..99 {
          }
          frame 100..199 {
          }
          frame 200..299 {
          }
          frame 300..399 {
          }
          frame 400..499 {
          }
          frame 500..599 {
          }
          frame 600..699 {
          }
          frame 700..799 {
          }
          frame 800..899 {
          }
          frame 900..999 {
          }
          frame 1000..1099 {
          }
          frame 1100..1199 {
          }
          frame 1200..1299 {
          }
          frame 1300..1399 {
          }
          frame 1400..1499 {
          }
          frame 1500..1599 {
          }
          frame 1600..1699 {
          }
          frame 1700..1799 {
          }
          frame 1800..1899 {
          }
          frame 1900..1999 {
          }
          frame 2000..2099 {
          }
          frame 2100..2199 {
          }
          frame 2200..2299 {
          }
          frame 2300..2399 {
          }
        }
        n128 = Bundle By Name(cluster=w687, "Year Code"=w684) -> (w685:T4)
        n129 = call <vilib>:"Add State(s) to Queue__JKI_lib_State_Machine.vi"("State(s) in (\"\")"=w690) -> ("States Out"=w689:string)  [unwired: 14 in]
      }
    }
  }
  "error out" <- w1
